vi "CMD_EXEC.vi"(6 "Gantry Class in":refnum<class "Gantry.lvclass">, 7 "Console Log in":refnum<class "Console Log.lvclass">, 8 "error in (no error)":errorcluster, 10 "Arguments":string[](array[string]), 11 "gScript Interpreter in":refnum<class "gScript Interpreter.lvclass">) -> (0 "error out":errorcluster, 3 "gScript Interpreter out":refnum<class "gScript Interpreter.lvclass">, 4 "Gantry Class out":refnum<class "Gantry.lvclass">, 5 "Console Log out":refnum<class "Console Log.lvclass">)   [LabVIEW 2024, in "gScript Interpreter.lvclass"]
uses:
  gScript Interpreter.lvclass
  Application Utilities/Console Log/Console Log.lvclass
  Shared Components/Gantry Class/Gantry.lvclass
  gScript Interpreter.lvclass/gScript Interpreter.ctl
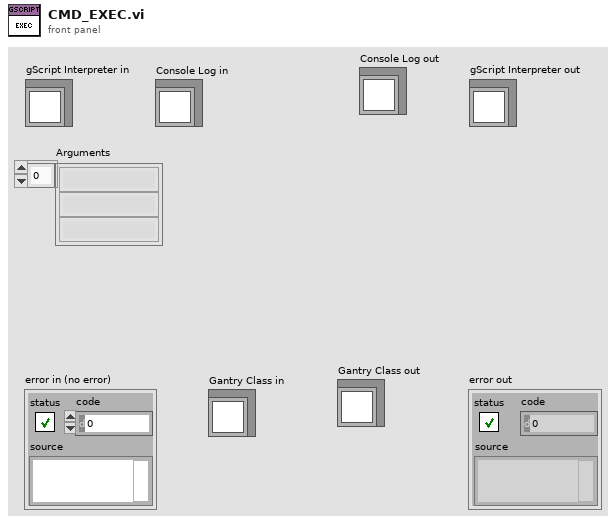
[diagram p1: front panel]
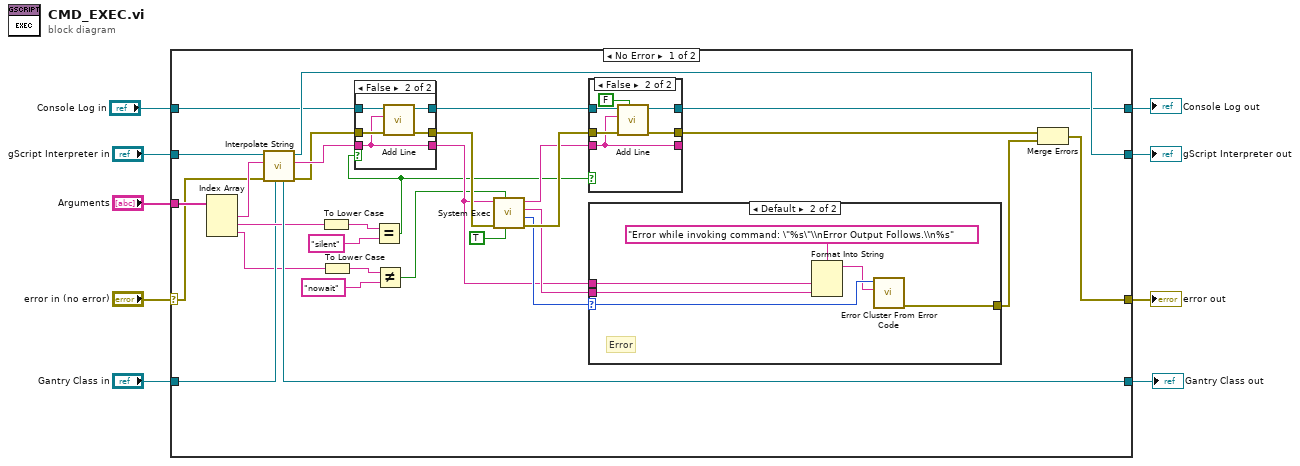
[diagram p0: block diagram]
diagram:
  n1 = case shown="No Error" "error in (no error)" {
    selector: "error in (no error)" -> [w37 w66]
    tunnel: [w18 w66] -> w8
    tunnel: [w35 w65] -> w6
    tunnel: "gScript Interpreter in" -> [w36 w65]
    tunnel: "Arguments" -> [w39 _]
    tunnel: "Console Log in" -> [w30 w64]
    tunnel: [w21 w64] -> w3
    tunnel: "Gantry Class in" -> [w16 w63]
    tunnel: [w34 w63] -> w1
    frame No Error {
      n2 = Index Array(array=w39) -> (element #1=w38:string, element #2=w33:string, element #3=w11:string)  [unwired: 3 in]
      n3 = call-dynamic "Interpolate String.vi"("Gantry in"=w16, "error in (no error)"=w37, "Input String"=w38, "gScript Interpreter in"=w36) -> ("error out"=w28:errorcluster, "Output String"=w29:string, "gScript Interpreter out"=w35:refnum<class "gScript Interpreter.lvclass">, "Gantry out"=w34:refnum<class "Gantry.lvclass">)  [unwired: 4 in]
      n4 = To Lower Case(string=w33) -> (all lower case string=w32:string)
      n5 = To Lower Case(string=w11) -> (all lower case string=w13:string)
      n6 = Equal?(x=w32, y="silent") -> (x = y?=w14:bool)
      n7 = case shown="False" w14 {
        tunnel: w30 -> [w57 w62]
        tunnel: w29 -> [w56 w59]
        tunnel: [w57 w61] -> w26
        tunnel: w28 -> [w55 w60]
        tunnel: [w56 w59] -> w17
        tunnel: [w55 w58] -> w27
        frame True {
        }
        frame False {
          n8 = call "Add Line.vi"("error in"=w60, "String"=w59, "Console Log in"=w62) -> ("error out"=w58:errorcluster, "Console Log out"=w61:refnum<class "Console Log.lvclass">)  [unwired: 7 in]
        }
      }
      n9 = Not Equal?(x=w13, y="nowait") -> (x != y?=w10:bool)
      n10 = call <vilib>:"System Exec.vi"("run minimized? (F)"=TRUE, "wait until completion? (T)"=w10, "error in (no error)"=w27, "command line"=w17) -> ("error out"=w25:errorcluster, "return code"=w22:i32, "standard error"=w23:string, "standard output"=w24:string)  [unwired: 4 in]
      n11 = case shown="False" w14 {
        tunnel: w26 -> [w48 w54]
        tunnel: w24 -> [w47 w51]
        tunnel: [w48 w53] -> w21
        tunnel: w25 -> [w46 w52]
        tunnel: [w47 w51] -> _
        tunnel: [w46 w50] -> w20
        frame True {
        }
        frame False {
          n12 = call "Add Line.vi"("Timestamp"=FALSE, "error in"=w52, "String"=w51, "Console Log in"=w54) -> ("error out"=w50:errorcluster, "Console Log out"=w53:refnum<class "Console Log.lvclass">)  [unwired: 6 in]
        }
      }
      n13 = case shown="Default" w22 {
        selector: w22 -> [_ w45]
        tunnel: w23 -> [_ w42]
        tunnel: [_ w43] -> w19
        tunnel: w17 -> [_ w41]
        frame 0 {
          # "Success"
        }
        frame Default {
          # "Error"
          n14 = Format Into String(format string="Error while invoking command: \"%s\"\\nError Output Follows.\\n%s", w41, w42) -> (resulting string=w40:string)  [unwired: 2 in, 1 out]
          n15 = call <vilib>:"Error Cluster From Error Code.vi"("error message (\"\")"=w40, "error code (0)"=w45) -> ("error out"=w43:errorcluster)  [unwired: 7 in]
        }
      }
      n16 = Merge Errors(w20, w19) -> (w18:errorcluster)
    }
    frame Error {
    }
  }
  "error out" <- w8
  "gScript Interpreter out" <- w6
  "Console Log out" <- w3
  "Gantry Class out" <- w1
